vi "GetRxPendingMsg.vi"(8 "error in (no error)":errorcluster, 11 "GenericCanAdapterClass in":refnum<class "GenericCanAdapterClass.lvclass">) -> (0 "error out":errorcluster, 2 "Value":i32, 3 "GenericCanAdapterClass out":refnum<class "GenericCanAdapterClass.lvclass">)   [LabVIEW 2011, in "GenericCanAdapterClass.lvclass"]
uses:
  GenericCanAdapterClass.lvclass
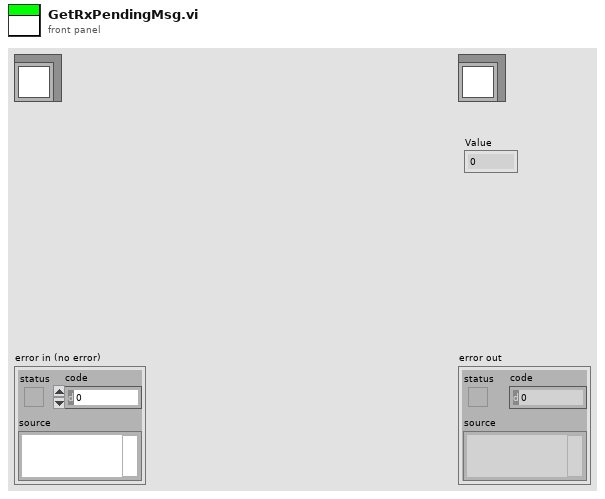
[diagram p1: front panel]
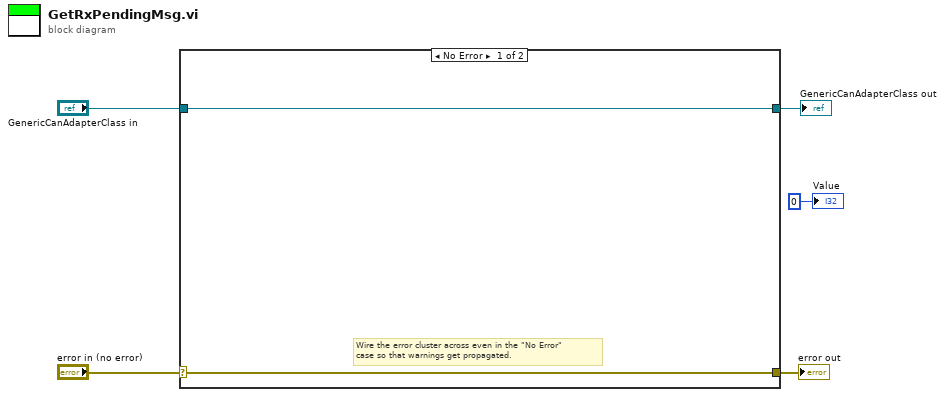
[diagram p0: block diagram]
diagram:
  n1 = case shown="No Error" "error in (no error)" {
    selector: "error in (no error)" -> [w6 w9]
    tunnel: [w6 w9] -> w4
    tunnel: [w7 w8] -> w2
    tunnel: "GenericCanAdapterClass in" -> [w7 w8]
    frame No Error {
      # "Wire the error cluster across even in the \"No Error\"\ncase so that warnings get propagated."
    }
    frame Error {
    }
  }
  "error out" <- w4
  "GenericCanAdapterClass out" <- w2
  "Value" <- 0
